vi "DCS_Spot_Query.vi"(0 "Enable":bool=TRUE, 5 "error in (no error)":errorcluster) -> (14 "Spot":T1, 15 "Cancel loading":bool caption="Cancel", 18 "OK":bool, 19 "error out":errorcluster)   [LabVIEW 2013]
doc: "Displays a standard dialog box that prompts users to enter information, such as a user name and password.\n--------------------\n\nThis Express VI is configured as follows:\n\nMessage to Display to the User:\nThe inputs are: \nNumber: Upper Timestamp Range\nNumber: Lower Timestamp Range\nNumber: Settings ID"
uses:
  <userlib>/Accelerator/User Interface/Controls/DCSConstraints.ctl
  <userlib>/Accelerator/User Interface/Controls/Constraints.ctl
  <vilib>/Math Plots/3D Math Plots/3D Surface/3D Surface XCtrl/3D Surface.xctl
  <userlib>/Accelerator/User Interface/Controls/dcs_spot.ctl
  <vilib>/Math Plots/3D Math Plots/3D Surface/3D Surface Datatype/3D Surface Datatype.lvclass
panel:
  in  "experiment settings Okay":bool
  in  "experiment settings dropdown":bool
  out "Current Spot Timestamp:":timestamp
  out "Number of matching spots:":dbl
  in  "Current Spot ID:":i64(ring) items=["Any Spot"=-1]
  out "Orange Cursor Position":dbl[](array[numeric]) min=-12.0 max=12.0 step=0.1 format="%.3g"
  out "3D Surface":refnum<class "3D Plot Datatype.lvclass">[](xcontrol)
  in  "Constraints":T2={"Upper Timestamp Range"=timestamp(0 s since 1904-01-01), "Lower Timestamp Range"=timestamp(0 s since 1904-01-01), "Experiment Group:"="", "Experiment Name:"=[0], "name array"=[], "Dust Spot ID"=0.0}
  in  "OK2":bool
  in  "Cancel":bool
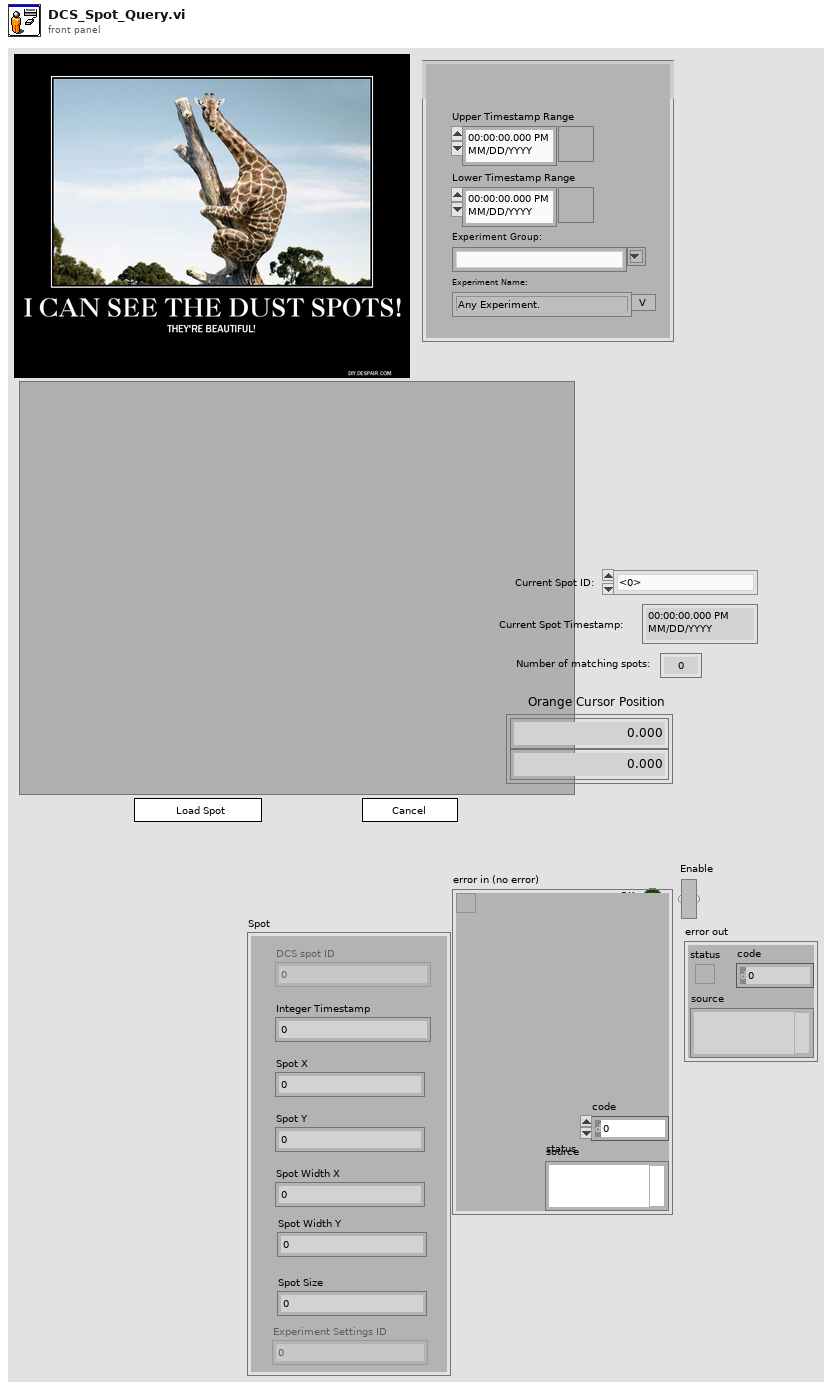
[diagram p1: front panel]
types:
  T1 = typedef "dcs_spot.ctl" = cluster{"DCS spot ID":i32, "Integer Timestamp":i64, "Spot X":dbl, "Spot Y":dbl, "Spot Width X":dbl, "Spot Width Y":dbl, "Spot Size":i32, "Experiment Settings ID":i32}
  T2 = typedef "DCSConstraints.ctl" = cluster{"Upper Timestamp Range":timestamp, "Lower Timestamp Range":timestamp, "Experiment Group:":string, "Experiment Name:":i32[], "name array":string[], "Dust Spot ID":dbl}
  T3 = typedef "Constraints.ctl" = cluster{"Upper Timestamp Range":timestamp, "Lower Timestamp Range":timestamp, "Experiment Group:":string, "Experiment Name:":i32[], "Upper Velocity Limit (km/s)":dbl, "Lower Velocity Limit (km/s)":dbl, "Upper Mass Limit (kg)":dbl, "Lower Mass Limit (kg)":dbl, "name array":string[], "Estimate Quality":cluster{dbl, dbl}}
  T4 = typedef "3D Plot.lvclass/Cursor Property Array.ctl" = T5[]
  T5 = typedef "3D Plot.lvclass/Cursor Property.ctl" = cluster{"Cursor Visible":bool, "Cursor Enable":bool, "Cursor Position":T6, "Cursor Point":T7, "Cursor Line":T9, "Cursor Plane":T11, "Cursor Text":T12}
  T6 = typedef "3D Plot.lvclass/Cursor Position.ctl" = cluster{"Cursor Plot ID":i32, "Cursor X":sgl, "Cursor Y":sgl, "Cursor Z":sgl, "Cursor Snap To":enum16{"Fixed", "Nearest Plot", "Snap to Plot"}}
  T7 = typedef "3D Plot.lvclass/Cursor Point.ctl" = cluster{"Cursor Point Color":u32, "Cursor Point Size":sgl, "Cursor Point Style":T8}
  T8 = typedef "3D Plot.lvclass/Sprite Type.ctl" = enum16{"None", "Empty Square", "Solid Square", "Empty Diamond", "Solid Diamond", "Empty Circle", "Solid Circle", "Asterisk", "Bold X", "Wireframe Sphere", "Solid Sphere", "Wireframe Cube", "Solid Cube"}
  T9 = typedef "3D Plot.lvclass/Cursor Line.ctl" = cluster{"Cursor Line Color":u32, "Cursor Line Width":sgl, "Cursor Line Style":T10}
  T10 = typedef "3D Plot.lvclass/Line Type.ctl" = enum16{"None", "Solid", "Dash", "Dot", "Dash Dot"}
  T11 = typedef "3D Plot.lvclass/Cursor Plane.ctl" = cluster{"Cursor Plane Color":u32, "Cursor Plane Opacity":sgl, "Draw Cursor Plane X-Z":bool, "Draw Cursor Plane Y-Z":bool, "Draw Cursor Plane X-Y":bool}
  T12 = typedef "3D Plot.lvclass/Cursor Text.ctl" = cluster{"Cursor Text":string, "Cursor Text Size":u16, "Cursor Show Position":bool, "Cursor Show Name":bool, "Cursor Text Color":u32, "Background Color":u32, "Background Opacity":sgl}
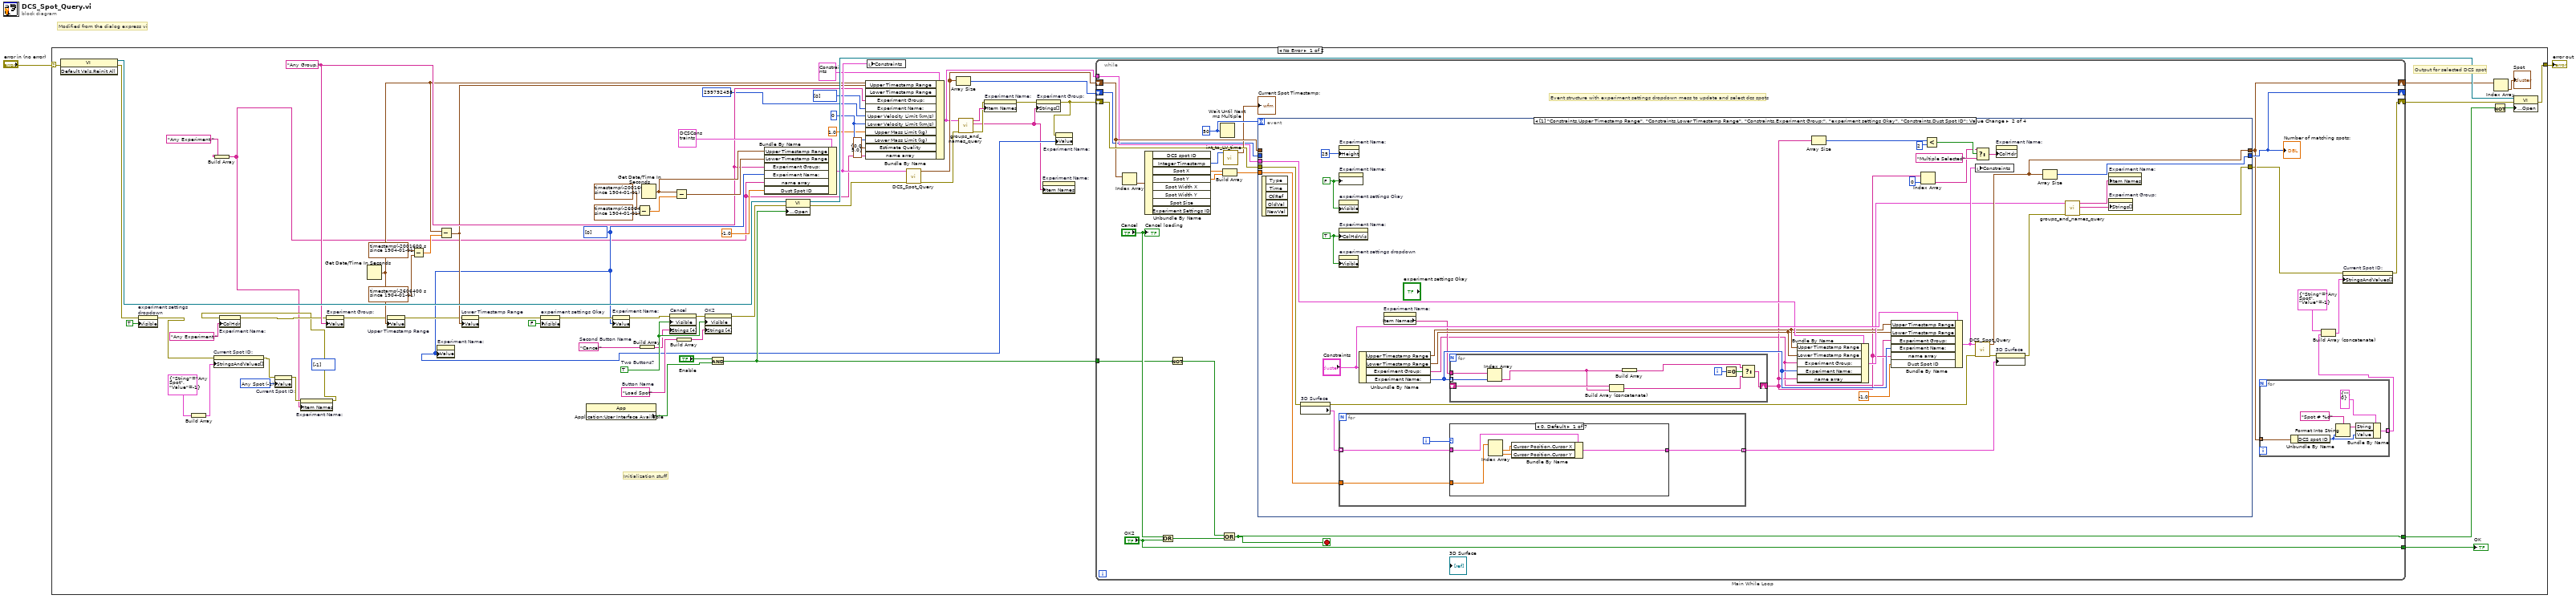
[diagram p0: block diagram]
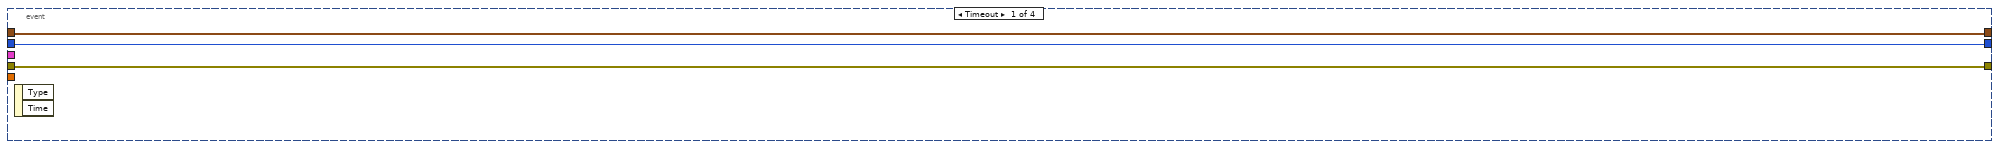
[diagram p2: hidden frame]
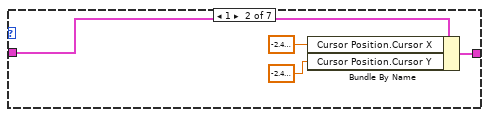
[diagram p3: hidden frame]
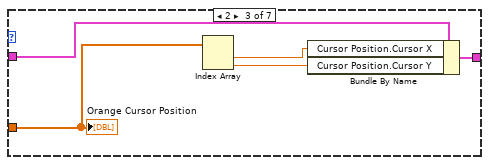
[diagram p4: hidden frame]
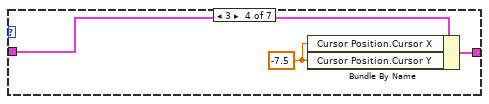
[diagram p5: hidden frame]
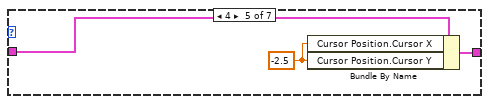
[diagram p6: hidden frame]
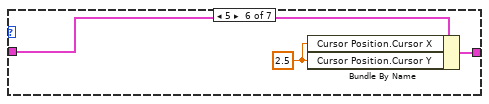
[diagram p7: hidden frame]
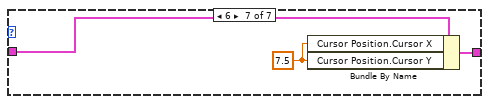
[diagram p8: hidden frame]
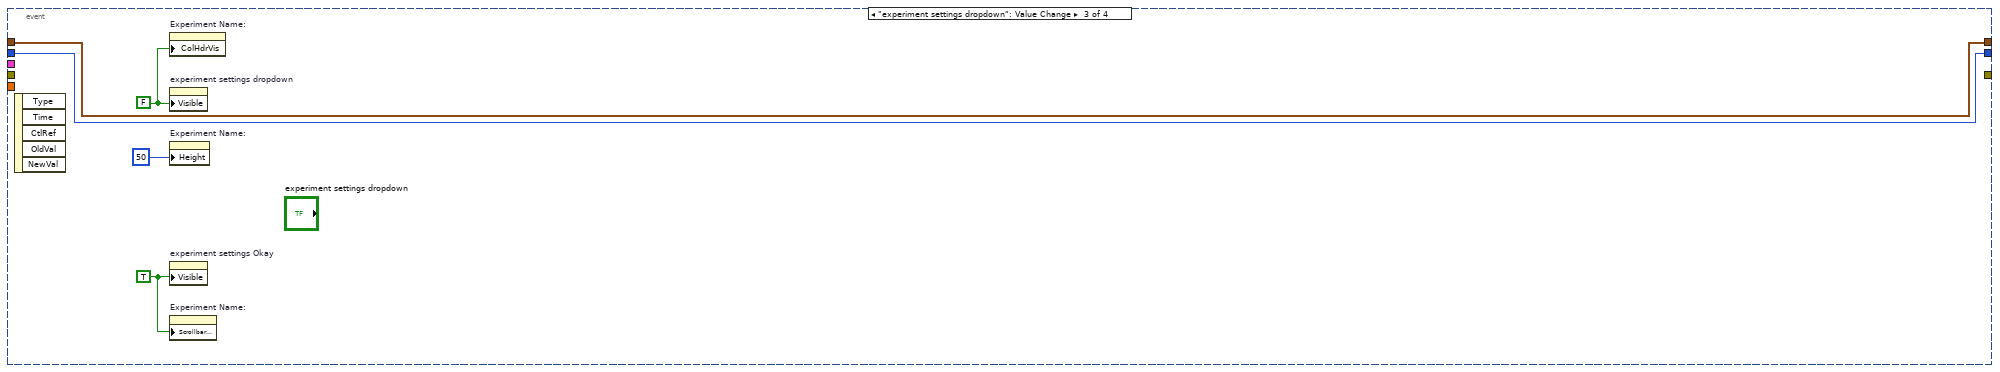
[diagram p9: hidden frame]
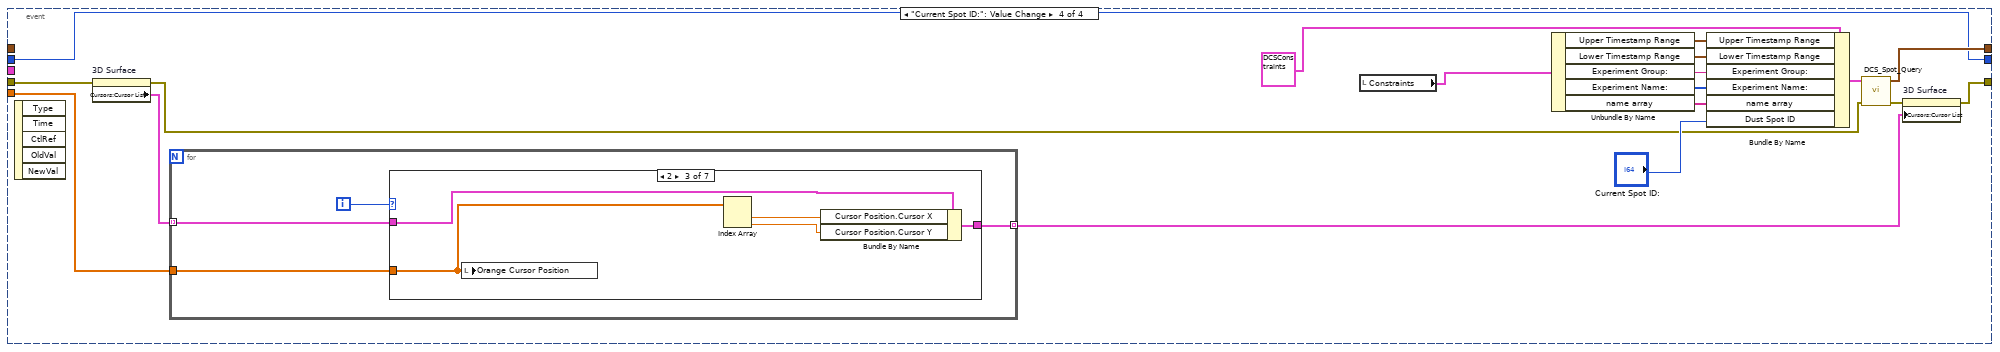
[diagram p10: hidden frame]
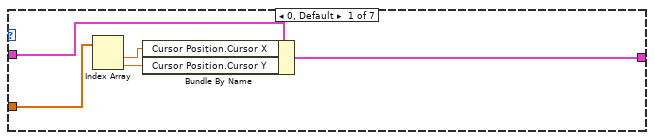
[diagram p11: hidden frame]
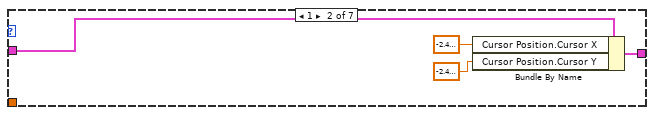
[diagram p12: hidden frame]
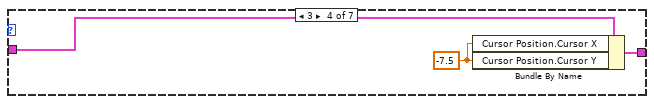
[diagram p13: hidden frame]
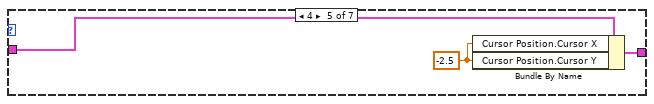
[diagram p14: hidden frame]
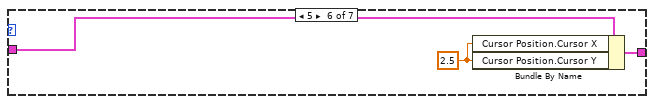
[diagram p15: hidden frame]
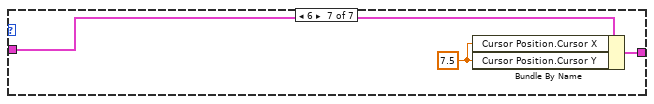
[diagram p16: hidden frame]
diagram:
  # "Modified from the dialog express vi"
  n1 = case shown="No Error" "error in (no error)" {
    selector: "error in (no error)" -> [w25 w231]
    tunnel: [w62 w231] -> w2
    frame No Error {
      (unwired) i32[] [-1] ("Value")
      w13 = i64 -1 items=["Any Spot"=-1, "Spot # 232"=232, "Spot # 233"=233, "Spot # 234"=234, "Spot # 235"=235, "Spot # 236"=236, "Spot # 237"=237, "Spot # 238"=238, "Spot # 239"=239, "Spot # 240"=240] ("Current Spot ID:")
      w38 = i64 0 ("Lower Timestamp Limit")
      w36 = "Any Group." ("element")
      w10 = i32[] [0] ("Experiment Name:")
      w66 = "Cancel"  # Second Button Name
      w64 = "Load Spot"  # Button Name
      w72 = TRUE  # Two Buttons?
      # "Output for selected DCS spot"
      # "Initialization stuff"
      n2 = invoke class="VI" method="Default Vals.Reinit All"(error in=w25) -> (reference out=w59:refnum<vi>, error out=w24:errorcluster)  [unwired: 2 in, 1 out]
      n3 = property on="experiment settings dropdown" class="Bool (strict)"(error in=w24, "Visible"=TRUE) -> (error out=w14:errorcluster)  [unwired: 1 in, 1 out]
      n4 = Build Array(cluster{"String":string, "Value":i64} {"String"="Any Spot", "Value"=-1} ("element")) -> (w15:cluster{"String":string, "Value":i64}[])
      n5 = property on="Current Spot ID:" class="Ring (strict)"(error in=w14, "StringsAndValues[]"=w15) -> (error out=w12:errorcluster)  [unwired: 1 in, 1 out]
      n6 = Build Array("Any Experiment." ("element")) -> (w4:string[])
      n7 = property on="Current Spot ID:" class="Ring (strict)"(error in=w12, "Value"=w13) -> (error out=w7:errorcluster)  [unwired: 1 in, 1 out]
      n8 = property on="Experiment Name:" class="LstBox (strict)"(error in=w7, "Item Names"=w4) -> (error out=w6:errorcluster)  [unwired: 1 in, 1 out]
      n9 = property on="Experiment Name:" class="LstBox (strict)"(error in=w6, "ColHdr"="Any Experiment." ("element")) -> (error out=w8:errorcluster)  [unwired: 1 in, 1 out]
      n10 = property on="Experiment Group:" class="CmbBox"(error in=w8, "Value"=w36) -> (error out=w23:errorcluster)  [unwired: 1 in, 1 out]
      n11 = Get Date/Time In Seconds() -> (seconds since 1Jan1904=w30:timestamp)
      n12 = property on="Upper Timestamp Range" class="AbsTime (strict)"(error in=w23, "Value"=w30) -> (error out=w22:errorcluster)  [unwired: 1 in, 1 out]
      n13 = Subtract(x=timestamp(-2001600 s since 1904-01-01) ("current time"), y=timestamp(-2606400 s since 1904-01-01) ("current time")) -> (x-y=w40:dbl)
      n14 = property on="Experiment Name:" class="LstBox (strict)"("Value"=w10) -> ()  [unwired: 2 in, 2 out]
      n15 = Subtract(x=w30, y=w40) -> (x-y=w29:timestamp)
      n16 = property on="Lower Timestamp Range" class="AbsTime (strict)"(error in=w22, "Value"=w29) -> (error out=w20:errorcluster)  [unwired: 1 in, 1 out]
      n17 = property on="experiment settings Okay" class="Bool (strict)"(error in=w20, "Visible"=FALSE) -> (error out=w19:errorcluster)  [unwired: 1 in, 1 out]
      n18 = property class="App"() -> ("Application:User Interface Available"=w60:bool)  [unwired: 2 in, 2 out]
      n19 = property on="Experiment Name:" class="LstBox (strict)"(error in=w19, "Value"=w10) -> (error out=w21:errorcluster)  [unwired: 1 in, 1 out]
      n20 = Subtract(x=timestamp(-2001600 s since 1904-01-01) ("Lower Timestamp Range"), y=timestamp(-2606400 s since 1904-01-01) ("Lower Timestamp Range")) -> (x-y=w55:dbl)
      n21 = Build Array(w66) -> (w67:string[])
      n22 = Get Date/Time In Seconds() -> (seconds since 1Jan1904=w51:timestamp)
      n23 = property on="Cancel" class="Bool"(error in=w21, "Visible"=w72, "Strings [4]"=w67) -> (error out=w70:errorcluster)  [unwired: 1 in, 1 out]
      n24 = Subtract(x=w51, y=w55) -> (x-y=w50:timestamp)
      n25 = Build Array(w64) -> (w65:string[])
      n26 = property on="OK2" class="Bool"(error in=w70, "Visible"=w72, "Strings [4]"=w65) -> (error out=w58:errorcluster)  [unwired: 1 in, 1 out]
      n27 = And(x="Enable", y=w60) -> (x .and. y?=w54:bool)
      n28 = Bundle By Name(cluster=T2 {"Upper Timestamp Range"=timestamp(0 s since 1904-01-01), "Lower Timestamp Range"=timestamp(0 s since 1904-01-01), "Experiment Group:"="", "Experiment Name:"=[], "name array"=[], "Dust Spot ID"=0.0} ("Constraints"), "Upper Timestamp Range"=w51, "Lower Timestamp Range"=w50, "Experiment Group:"=w36, "Experiment Name:"=w10, "name array"=w4, "Dust Spot ID"=-1.0) -> (w49:T2)
      n29 = property class="VI"(reference=w59, error in=w58, "Front Panel Window:Open"=w54) -> (reference out=w53:refnum<vi>, error out=w47:errorcluster)
      n30 = Bundle By Name(cluster=T3 {"Upper Timestamp Range"=timestamp(0 s since 1904-01-01), "Lower Timestamp Range"=timestamp(0 s since 1904-01-01), "Experiment Group:"="", "Experiment Name:"=[], "Upper Velocity Limit (km/s)"=0.0, "Lower Velocity Limit (km/s)"=0.0, "Upper Mass Limit (kg)"=0.0, "Lower Mass Limit (kg)"=0.0, "name array"=[], "Estimate Quality"={0.0, 0.0}} ("Constraints"), "Upper Timestamp Range"=w30, "Lower Timestamp Range"=w29, "Experiment Group:"=w36, "Experiment Name:"=i32[] [0], "Upper Velocity Limit (km/s)"=299792458, "Lower Velocity Limit (km/s)"=w38, "Upper Mass Limit (kg)"=1.0, "Lower Mass Limit (kg)"=w38, "Estimate Quality"=cluster{dbl, dbl} {0.0, 5.0}, "name array"=w4) -> (w31:T3)
      n31 = local write "Constraints"(w49) -> ()
      n32 = call <userlib>:"DCS_Spot_Query.vi"("error in (no error)"=w47, "Constraints"=w49) -> ("error out"=w32:errorcluster, "Array"=w46:T1[])  [unwired: 8 in]
      n33 = Array Size(array=w46) -> (size(s)=w45:i32)
      n34 = call <userlib>:"groups_and_names_query.vi"("error in (no error)"=w32, "Constraints"=w31) -> ("error out"=w18:errorcluster, "Groups"=w9:string[], "Names"=w33:string[])  [unwired: 5 in, 2 out]
      n35 = property on="Experiment Name:" class="LstBox (strict)"(error in=w18, "Item Names"=w33) -> (error out=w17:errorcluster)  [unwired: 1 in, 1 out]
      n36 = property on="Experiment Group:" class="CmbBox"(error in=w17, "Strings[]"=w9) -> (error out=w11:errorcluster)  [unwired: 1 in, 1 out]
      n37 = property on="Experiment Name:" class="LstBox (strict)"("Item Names"=w9) -> ()  [unwired: 2 in, 2 out]
      n38 = property on="Experiment Name:" class="LstBox (strict)"(error in=w11, "Value"=w10) -> ()  [unwired: 1 in, 2 out]
      n39 = while "Main While Loop" {
        tunnel: ["OK2"] -> w71
        tunnel: w54 -> [w95]
        tunnel: [w93] -> w68
        shift-right: [w76] -> w63
        shift-left: w11 -> [w90]
        shift-right: [w80] -> _
        shift-left: w45 -> [w79]
        shift-right: [w78] -> w44
        shift-left: w46 -> [w87]
        tunnel: w31 -> [w81]
        stop <- w93 stop-if-true
        w89 = u32 50 ("millisecond multiple")
        # "Event structure with experiment settings dropdown mess to update and select dcs spots"
        n40 = Index Array(array=w87) -> (element=w88:T1)  [unwired: 1 in]
        n41 = Unbundle By Name(w88) -> ("Integer Timestamp"=w85:i64, "Spot X"=w83:dbl, "Spot Y"=w82:dbl)  [unwired: 5 out]
        n42 = Or(x="Cancel", y="OK2") -> (x .or. y?=w92:bool)
        n43 = Not(x=w95) -> (.not. x?=w94:bool)
        n44 = Wait Until Next ms Multiple(millisecond multiple=w89) -> ()  [unwired: 1 out]
        n45 = Build Array(w83, w82) -> (w84:dbl[])
        n46 = call <userlib>:"int_to_LV_time.vi"("Integer Timestamp"=w85) -> ("time stamp"=→"Current Spot Timestamp:":timestamp)  [unwired: 8 in, 1 out]
        n47 = Compound Arithmetic op=OR(w94, w92) -> (w93:bool)
        n48 = event shown="[1] \"Constraints.Upper Timestamp Range\", \"Constraints.Lower Timestamp Range\", \"Constraints.Experiment Group:\", \"experiment settings Okay\", \"Constraints.Dust Spot ID\": Value Change" {
          selector: _ -> [_ _ _ _]
          dyn-events: _ -> [_ _ _ _]
          timeout: w89 -> [_ _ _ _]
          tunnel: w90 -> [w105 w136 _ w197]
          tunnel: [w105 w118 _ w198] -> w77
          tunnel: w79 -> [w104 _ w182 w187]
          tunnel: [w104 w135 w182 w187] -> w80
          tunnel: [w103 w131 w181 w188] -> w78
          tunnel: w87 -> [w103 _ w181 _]
          tunnel: w84 -> [_ w128 _ w184]
          tunnel: w81 -> [_ w125 _ _]
          event Timeout {
            n49 = event-data() -> ()  [unwired: 1 in, 2 out]
          }
          event "experiment settings Okay": Value Change {
            w117 = FALSE ("Visible")
            w116 = TRUE ("Visible")
            n50 = event-data() -> ()  [unwired: 1 in, 5 out]
            n51 = property on="3D Surface" class="3D Surface (strict)"(error in=w136) -> (error out=w130:errorcluster, "Cursors:Cursor List"=w137:T4)  [unwired: 1 in, 1 out]
            n52 = property on="Experiment Name:" class="LstBox (strict)"("Height"=u32 25 ("Size:Height")) -> ()  [unwired: 2 in, 2 out]
            n53 = property on="Experiment Name:" class="LstBox (strict)"("Scrollbar Visible"=w117) -> ()  [unwired: 2 in, 2 out]
            n54 = property on="experiment settings Okay" class="Bool (strict)"("Visible"=w117) -> ()  [unwired: 2 in, 2 out]
            n55 = property on="Experiment Name:" class="LstBox (strict)"("ColHdrVis"=w116) -> ()  [unwired: 2 in, 2 out]
            n56 = property on="experiment settings dropdown" class="Bool (strict)"("Visible"=w116) -> ()  [unwired: 2 in, 2 out]
            n57 = for {
              tunnel: w137 -> [w151] mode=indexing
              tunnel: [w149] -> w138 mode=indexing
              tunnel: w128 -> [w148]
              i -> [w150]
              n58 = case shown="0, Default" w150 {
                tunnel: w151 -> [w156 w159 w164 w168 w171 w174 w177]
                tunnel: [w155 w160 w165 w167 w170 w173 w176] -> w149
                tunnel: w148 -> [w154 _ w161 _ _ _ _]
                frame 0, Default {
                  n59 = Index Array(array=w154) -> (element #1=w153:dbl, element #2=w152:dbl)  [unwired: 2 in]
                  n60 = Bundle By Name(cluster=w156, "Cursor Position.Cursor X"=w153, "Cursor Position.Cursor Y"=w152) -> (w155:T5)
                }
                frame 1 {
                  n61 = Bundle By Name(cluster=w159, "Cursor Position.Cursor X"=sgl -2.4, "Cursor Position.Cursor Y"=sgl -2.4) -> (w160:T5)
                }
                frame 2 {
                  n62 = Index Array(array=w161) -> (element #1=w163:dbl, element #2=w162:dbl)  [unwired: 2 in]
                  n63 = Bundle By Name(cluster=w164, "Cursor Position.Cursor X"=w163, "Cursor Position.Cursor Y"=w162) -> (w165:T5)
                  "Orange Cursor Position" <- w161
                }
                frame 3 {
                  w166 = -7.5 ("index")
                  n64 = Bundle By Name(cluster=w168, "Cursor Position.Cursor X"=w166, "Cursor Position.Cursor Y"=w166) -> (w167:T5)
                }
                frame 4 {
                  w169 = -2.5 ("index")
                  n65 = Bundle By Name(cluster=w171, "Cursor Position.Cursor X"=w169, "Cursor Position.Cursor Y"=w169) -> (w170:T5)
                }
                frame 5 {
                  w172 = 2.5 ("index")
                  n66 = Bundle By Name(cluster=w174, "Cursor Position.Cursor X"=w172, "Cursor Position.Cursor Y"=w172) -> (w173:T5)
                }
                frame 6 {
                  w175 = 7.5 ("index")
                  n67 = Bundle By Name(cluster=w177, "Cursor Position.Cursor X"=w175, "Cursor Position.Cursor Y"=w175) -> (w176:T5)
                }
              }
            }
            n68 = Unbundle By Name("Constraints") -> ("Upper Timestamp Range"=w124:timestamp, "Lower Timestamp Range"=w123:timestamp, "Experiment Group:"=w106:string, "Experiment Name:"=w122:i32[])
            n69 = property on="Experiment Name:" class="LstBox (strict)"() -> ("Item Names"=w107:string[])  [unwired: 2 in, 2 out]
            n70 = for {
              tunnel: w122 -> [w146] mode=indexing
              tunnel: w107 -> [w147]
              shift-right: [w140] -> w108
              shift-left: _ -> [w141]
              i -> [w142]
              n71 = Index Array(array=w147, index=w146) -> (element=w139:string)
              n72 = Build Array (concatenate)(w141, w139) -> (w145:string[])
              n73 = Build Array(w139) -> (w144:string[])
              n74 = Equal To 0?(x=w142) -> (x = 0?=w143:bool)
              n75 = Select(t=w144, s=w143, f=w145) -> (s? t:f=w140:string[])
            }
            n76 = Bundle By Name(cluster=w125, "Upper Timestamp Range"=w124, "Lower Timestamp Range"=w123, "Experiment Group:"=w106, "Experiment Name:"=w122, "name array"=w108) -> (w126:T3)
            n77 = Array Size(array=w108) -> (size(s)=w113:i32)
            n78 = Bundle By Name(cluster="Constraints", "Upper Timestamp Range"=w124, "Lower Timestamp Range"=w123, "Experiment Group:"=w106, "Experiment Name:"=w122, "name array"=w108, "Dust Spot ID"=-1.0) -> (w132:T2)
            n79 = Index Array(array=w108, index=0) -> (element=w112:string)
            n80 = Less?(x=w113, y=2) -> (x < y?=w114:bool)
            n81 = Select(t=w112, s=w114, f="Multiple Selected") -> (s? t:f=w111:string)
            n82 = local write "Constraints"(w132) -> ()
            n83 = call <userlib>:"DCS_Spot_Query.vi"("error in (no error)"=w130, "Constraints"=w132) -> ("error out"=w129:errorcluster, "Array"=w131:T1[])  [unwired: 8 in]
            n84 = property on="Experiment Name:" class="LstBox (strict)"("ColHdr"=w111) -> ()  [unwired: 2 in, 2 out]
            n85 = property on="3D Surface" class="3D Surface (strict)"(error in=w129, "Cursors:Cursor List"=w138) -> (error out=w119:errorcluster)  [unwired: 1 in, 1 out]
            n86 = Array Size(array=w131) -> (size(s)=w135:i32)
            n87 = call <userlib>:"groups_and_names_query.vi"("error in (no error)"=w119, "Constraints"=w126) -> ("error out"=w118:errorcluster, "Groups"=w120:string[], "Names"=w121:string[])  [unwired: 5 in, 2 out]
            n88 = property on="Experiment Name:" class="LstBox (strict)"("Item Names"=w121) -> ()  [unwired: 2 in, 2 out]
            n89 = property on="Experiment Group:" class="CmbBox"("Strings[]"=w120) -> ()  [unwired: 2 in, 2 out]
          }
          event "experiment settings dropdown": Value Change {
            w178 = TRUE ("Visible Items:Vertical Scrollbar Visible")
            w179 = FALSE ("Visible Items:Vertical Scrollbar Visible")
            n90 = event-data() -> ()  [unwired: 1 in, 5 out]
            n91 = property on="Experiment Name:" class="LstBox (strict)"("ColHdrVis"=w179) -> ()  [unwired: 2 in, 2 out]
            n92 = property on="experiment settings dropdown" class="Bool (strict)"("Visible"=w179) -> ()  [unwired: 2 in, 2 out]
            n93 = property on="Experiment Name:" class="LstBox (strict)"("Height"=50 ("x")) -> ()  [unwired: 2 in, 2 out]
            n94 = property on="experiment settings Okay" class="Bool (strict)"("Visible"=w178) -> ()  [unwired: 2 in, 2 out]
            n95 = property on="Experiment Name:" class="LstBox (strict)"("Scrollbar Visible"=w178) -> ()  [unwired: 2 in, 2 out]
          }
          event "Current Spot ID:": Value Change {
            n96 = event-data() -> ()  [unwired: 1 in, 5 out]
            n97 = property on="3D Surface" class="3D Surface (strict)"(error in=w197) -> (error out=w186:errorcluster, "Cursors:Cursor List"=w199:T4)  [unwired: 1 in, 1 out]
            n98 = for {
              tunnel: w199 -> [w204] mode=indexing
              tunnel: [w202] -> w200 mode=indexing
              tunnel: w184 -> [w201]
              i -> [w203]
              n99 = case shown="2" w203 {
                tunnel: w204 -> [w209 w212 w217 w221 w224 w227 w230]
                tunnel: [w208 w213 w218 w220 w223 w226 w229] -> w202
                tunnel: w201 -> [w207 _ w216 _ _ _ _]
                frame 0, Default {
                  n100 = Index Array(array=w207) -> (element #1=w206:dbl, element #2=w205:dbl)  [unwired: 2 in]
                  n101 = Bundle By Name(cluster=w209, "Cursor Position.Cursor X"=w206, "Cursor Position.Cursor Y"=w205) -> (w208:T5)
                }
                frame 1 {
                  n102 = Bundle By Name(cluster=w212, "Cursor Position.Cursor X"=sgl -2.4, "Cursor Position.Cursor Y"=sgl -2.4) -> (w213:T5)
                }
                frame 2 {
                  n103 = local write "Orange Cursor Position"(w216) -> ()
                  n104 = Index Array(array=w216) -> (element #1=w215:dbl, element #2=w214:dbl)  [unwired: 2 in]
                  n105 = Bundle By Name(cluster=w217, "Cursor Position.Cursor X"=w215, "Cursor Position.Cursor Y"=w214) -> (w218:T5)
                }
                frame 3 {
                  w219 = -7.5 ("index")
                  n106 = Bundle By Name(cluster=w221, "Cursor Position.Cursor X"=w219, "Cursor Position.Cursor Y"=w219) -> (w220:T5)
                }
                frame 4 {
                  w222 = -2.5 ("index")
                  n107 = Bundle By Name(cluster=w224, "Cursor Position.Cursor X"=w222, "Cursor Position.Cursor Y"=w222) -> (w223:T5)
                }
                frame 5 {
                  w225 = 2.5 ("index")
                  n108 = Bundle By Name(cluster=w227, "Cursor Position.Cursor X"=w225, "Cursor Position.Cursor Y"=w225) -> (w226:T5)
                }
                frame 6 {
                  w228 = 7.5 ("index")
                  n109 = Bundle By Name(cluster=w230, "Cursor Position.Cursor X"=w228, "Cursor Position.Cursor Y"=w228) -> (w229:T5)
                }
              }
            }
            n110 = local read "Constraints"() -> (w190:T2)
            n111 = Unbundle By Name(w190) -> ("Upper Timestamp Range"=w192:timestamp, "Lower Timestamp Range"=w193:timestamp, "Experiment Group:"=w194:string, "Experiment Name:"=w196:i32[], "name array"=w195:string[])
            n112 = Bundle By Name(cluster=T2 {"Upper Timestamp Range"=timestamp(0 s since 1904-01-01), "Lower Timestamp Range"=timestamp(0 s since 1904-01-01), "Experiment Group:"="", "Experiment Name:"=[], "name array"=[], "Dust Spot ID"=0.0} ("Constraints"), "Upper Timestamp Range"=w192, "Lower Timestamp Range"=w193, "Experiment Group:"=w194, "Experiment Name:"=w196, "name array"=w195, "Dust Spot ID"="Current Spot ID:") -> (w189:T2)
            n113 = call <userlib>:"DCS_Spot_Query.vi"("error in (no error)"=w186, "Constraints"=w189) -> ("error out"=w185:errorcluster, "Array"=w188:T1[])  [unwired: 8 in]
            n114 = property on="3D Surface" class="3D Surface (strict)"(error in=w185, "Cursors:Cursor List"=w200) -> (error out=w198:errorcluster)  [unwired: 1 in, 1 out]
          }
        }
        "Number of matching spots:" <- w80
        n115 = for {
          tunnel: w78 -> [w102] mode=indexing
          tunnel: [w100] -> w74 mode=indexing
          n116 = Unbundle By Name(w102) -> ("DCS spot ID"=w98:i32)
          n117 = Format Into String(format string="Spot # %d", w98) -> (resulting string=w99:string)  [unwired: 2 in, 1 out]
          n118 = Bundle By Name(cluster=cluster{"String":string, "Value":i64} {"String"="", "Value"=0} ("element"), "String"=w99, "Value"=w98) -> (w100:cluster{"String":string, "Value":i64})
        }
        n119 = Build Array (concatenate)(cluster{"String":string, "Value":i64} {"String"="Any Spot", "Value"=-1} ("element"), w74) -> (w75:cluster{"String":string, "Value":i64}[])
        n120 = property on="Current Spot ID:" class="Ring (strict)"(error in=w77, "StringsAndValues[]"=w75) -> (error out=w76:errorcluster)  [unwired: 1 in, 1 out]
        "Cancel loading" <- "Cancel"
      }
      "OK" <- w71
      n121 = Not(x=w68) -> (.not. x?=w69:bool)
      n122 = Index Array(array=w44) -> (element=→"Spot":T1)  [unwired: 1 in]
      n123 = property class="VI"(reference=w53, error in=w63, "Front Panel Window:Open"=w69) -> (error out=w62:errorcluster)  [unwired: 1 out]
    }
    frame Error {
    }
  }
  "error out" <- w2
